vi "Add Points.vi"(7 "no of points":u8, 8 "error in (no error)":errorcluster, 10 "Identifier":u32, 11 "Item Ref in":T1=18446744073709551615 format="%.0x") -> (0 "error out":errorcluster, 3 "Item Ref out":T1=18446744073709551615 format="%.0x")   [LabVIEW 2023, in "Vires VTD System Explorer.lvlib"]
uses:
  Vires VTD System Explorer.lvlib
  <vilib>/NI VeriStand/Custom Device API/Custom Device Item Ref.ctl
  Shared/Constants.vi
  <vilib>/NI VeriStand/Custom Device API/Custom Device API.lvlib
  Shared/Vires VTD Shared.lvlib
panel:
  in  "PlayerID":u8
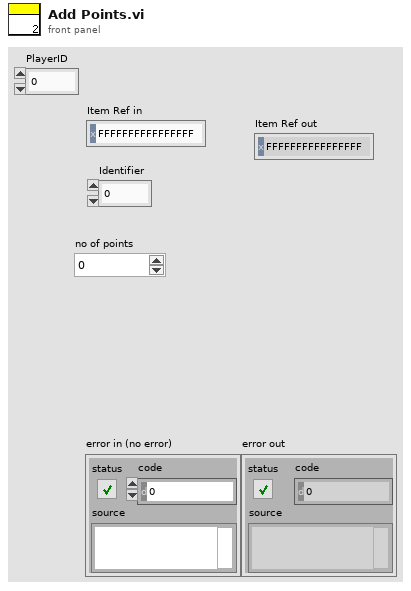
[diagram p1: front panel]
types:
  T1 = typedef "Custom Device API.lvlib/Custom Device Item Ref.ctl" = u64
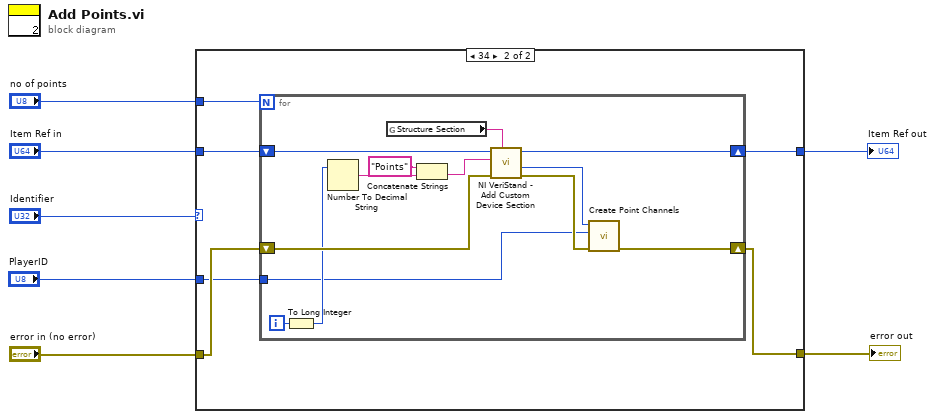
[diagram p0: block diagram]
diagram:
  n1 = case shown="34" "Identifier" {
    tunnel: "Item Ref in" -> [w9 w15]
    tunnel: [w9 w14] -> w5
    tunnel: "error in (no error)" -> [w8 w12]
    tunnel: [w8 w13] -> w3
    tunnel: "no of points" -> [_ w11]
    tunnel: "PlayerID" -> [_ w10]
    frame Default {
    }
    frame 34 {
      n2 = for {
        N: w11 -> [_]
        shift-right: [w20] -> w14
        shift-left: w15 -> [w28]
        shift-right: [w17] -> w13
        shift-left: w12 -> [w27]
        tunnel: w10 -> [w16]
        i -> [w21]
        n3 = To Long Integer(number=w21) -> (32bit integer=w23:i32)
        n4 = Number To Decimal String(number=w23) -> (decimal integer string=w25:string)  [unwired: 1 in]
        n5 = global read "Constants.vi" "Structure Section"() -> (w22:string)
        n6 = Concatenate Strings("Points" ("string"), w25) -> (w24:string)
        n7 = call <vilib>:"NI VeriStand - Add Custom Device Section.vi"("GUID (Default Section)"=w22, "error in (no error)"=w27, "Section Name"=w24, "Parent Ref in"=w28) -> ("error out"=w18:errorcluster, "Section Ptr"=w19:T1, "Parent Ref out"=w20:T1)  [unwired: 4 in, 1 out]
        n8 = call "Create Point Channels.vi"("error in (no error)"=w18, "PlayerID"=w16, "Parent Ref in"=w19) -> ("error out"=w17:errorcluster)  [unwired: 7 in, 1 out]
      }
    }
  }
  "error out" <- w3
  "Item Ref out" <- w5
